vi "Test Platine newport.vi"() -> ()   [LabVIEW 2024]
uses:
  Newport.SMC100.CommandInterface
panel:
  in  "Init":bool
  out "Etat Controleur":bool
  out "StageIdentifier":string
  in  "Set Pos.Abs":bool
  in  "RESET Ctrl":bool
  in  "TargetPosition Abs":dbl
  out "Get PA Position":dbl
  out "Open Error":i32
  out "controllerState":string
  out "Close Error":i32
  in  "Controller address":i32=1
  out "CurrentPosition":dbl
  out "TS error":i32
  out "TP error":i32
  out "VE error":i32
  out "Error out":errorcluster caption="error out"
  in  "COM Port":string
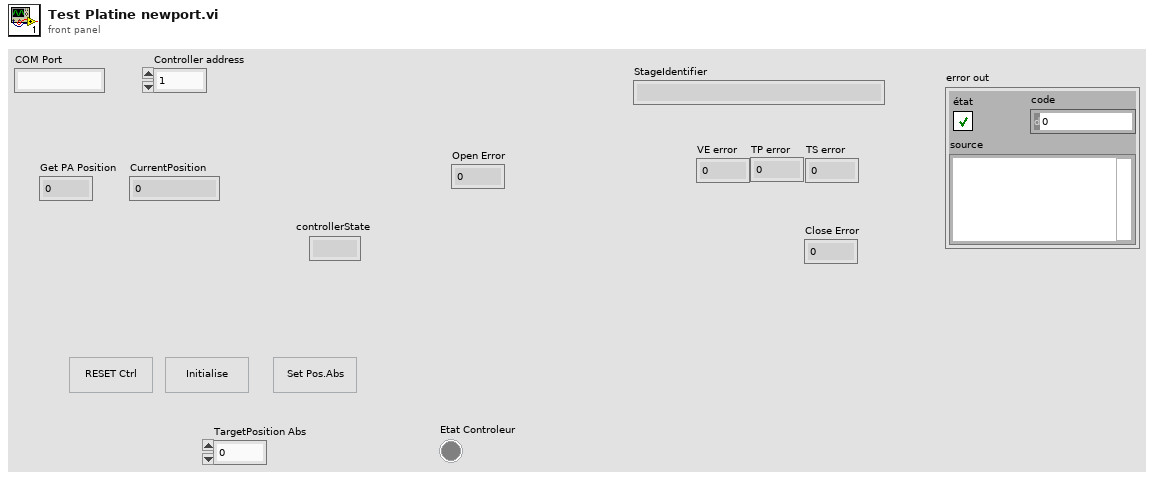
[diagram p1: front panel]
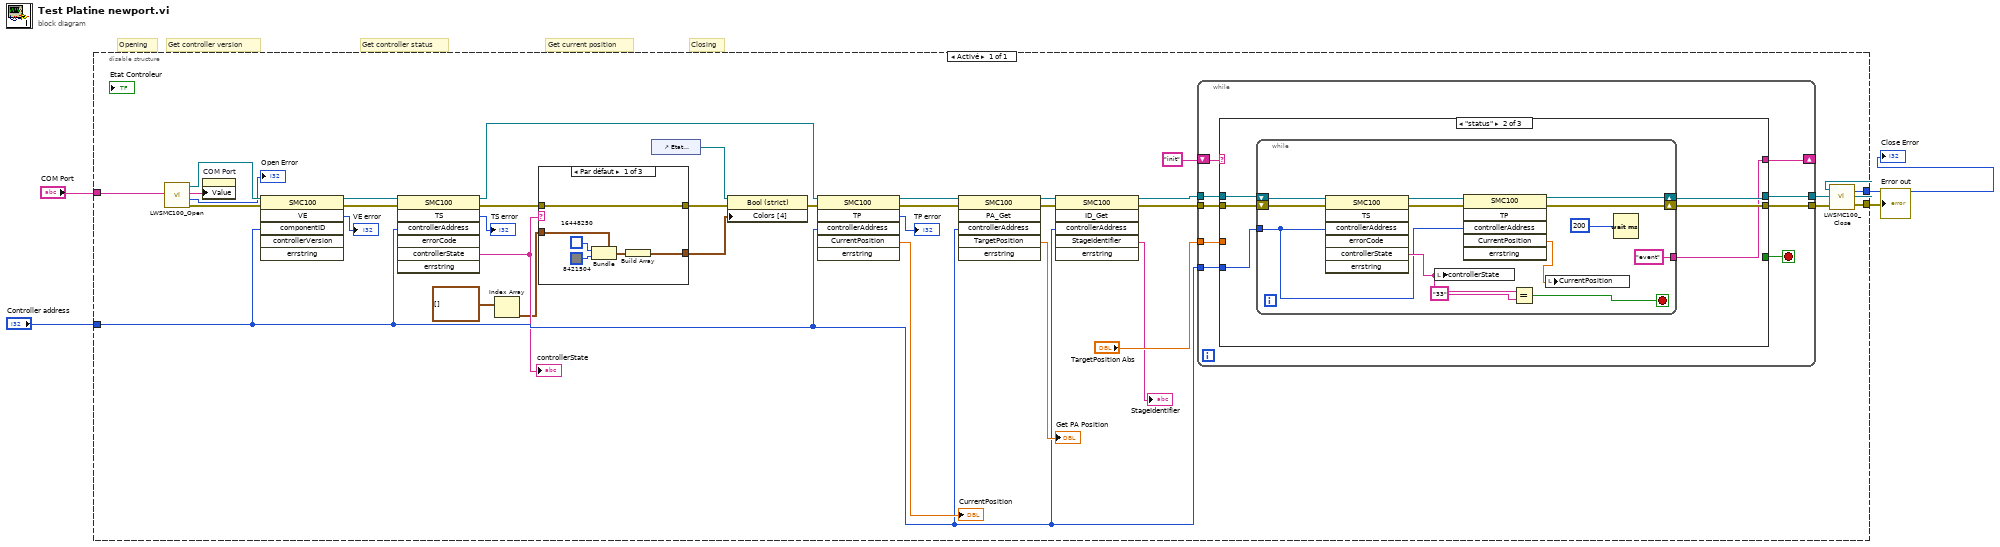
[diagram p0: block diagram]
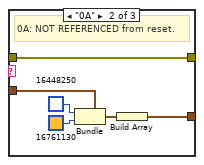
[diagram p2: hidden frame]
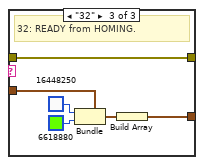
[diagram p3: hidden frame]
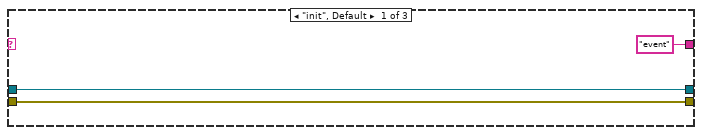
[diagram p4: hidden frame]
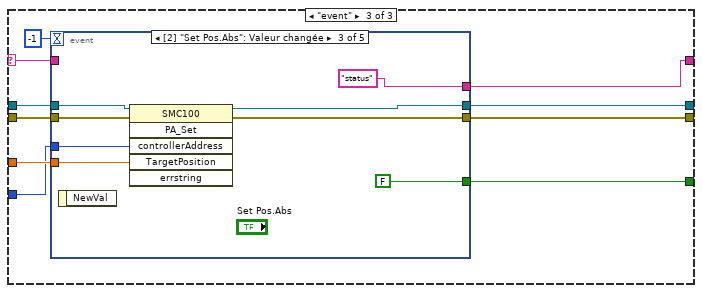
[diagram p5: hidden frame]
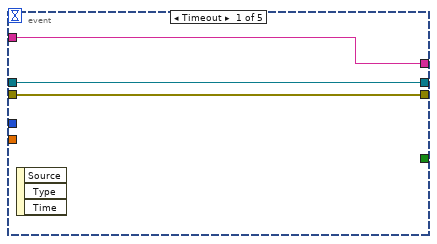
[diagram p6: hidden frame]
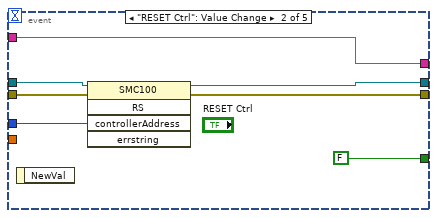
[diagram p7: hidden frame]
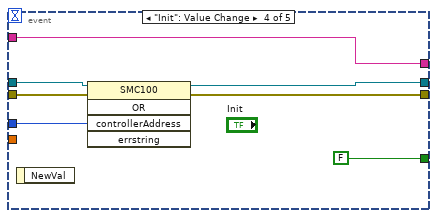
[diagram p8: hidden frame]
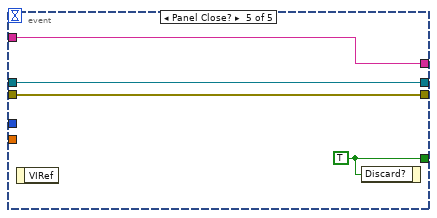
[diagram p9: hidden frame]
diagram:
  # "Get controller status"
  # "Get controller version"
  # "Get current position"
  # "Closing"
  # "Opening"
  n1 = disable-structure shown="Activé" {
    disable-tunnel: [w39] -> w4
    disable-tunnel: "COM Port" -> [w32]
    disable-tunnel: [w27] -> w2
    disable-tunnel: "Controller address" -> [w15]
    frame Enabled {
      n2 = call "LWSMC100_Open.vi"("Instrument Key IN"=w32) -> ("error out"=w31:errorcluster, "Error"=→"Open Error":i32, "Instrument Key OUT"=w33:string, "CommandInterfaceSMC100.SMC100"=w30:refnum<k24>)  [unwired: 3 in]
      n3 = property on="COM Port" class="Ch"("Value"=w33) -> ()  [unwired: 2 in, 2 out]
      n4 = invoke class="SMC100" method="VE"(reference=w30, error in=w31, "componentID"=w15) -> (reference out=w34:refnum<k24>, error out=w29:errorcluster, "VE"=→"VE error":i32)  [unwired: 3 in, 3 out]
      n5 = invoke class="SMC100" method="TS"(reference=w34, error in=w29, "controllerAddress"=w15) -> (reference out=w36:refnum<k24>, error out=w11:errorcluster, "TS"=→"TS error":i32, "controllerState"=w12:string)  [unwired: 4 in, 3 out]
      "controllerState" <- w12
      n6 = Index Array(array=cluster{u32, u32}[] [] ("Couls [4]")) -> (element=w9:cluster{u32, u32})  [unwired: 1 in]
      n7 = case shown="Par défaut" w12 {
        tunnel: w11 -> [w45 w51 w57]
        tunnel: [w45 w51 w57] -> w7
        tunnel: w9 -> [w41 w48 w54]
        tunnel: [w40 w46 w52] -> w8
        frame Default {
          n8 = Bundle(cluster=w41, u32 16448250, u32 8421504) -> (w42:cluster{u32, u32})
          n9 = Build Array(w42) -> (w40:cluster{u32, u32}[])
        }
        frame "0A" {
          # "0A: NOT REFERENCED from reset."
          n10 = Bundle(cluster=w48, u32 16448250, u32 16761130) -> (w47:cluster{u32, u32})
          n11 = Build Array(w47) -> (w46:cluster{u32, u32}[])
        }
        frame "32" {
          # "32: READY from HOMING."
          n12 = Bundle(cluster=w54, u32 16448250, u32 6618880) -> (w53:cluster{u32, u32})
          n13 = Build Array(w53) -> (w52:cluster{u32, u32}[])
        }
      }
      n14 = control-ref of="Etat Controleur"() -> (w13:refnum<vi>)
      n15 = property class="Bool (strict)"(reference=w13, error in=w7, "Colors [4]"=w8) -> (error out=w6:errorcluster)  [unwired: 1 out]
      n16 = invoke class="SMC100" method="TP"(reference=w36, error in=w6, "controllerAddress"=w15) -> (reference out=w24:refnum<k24>, error out=w25:errorcluster, "TP"=→"TP error":i32, "CurrentPosition"=→"CurrentPosition":dbl)  [unwired: 3 in, 2 out]
      n17 = invoke class="SMC100" method="PA_Get"(reference=w24, error in=w25, "controllerAddress"=w15) -> (reference out=w22:refnum<k24>, error out=w21:errorcluster, "TargetPosition"=→"Get PA Position":dbl)  [unwired: 3 in, 3 out]
      n18 = invoke class="SMC100" method="ID_Get"(reference=w22, error in=w21, "controllerAddress"=w15) -> (reference out=w19:refnum<k24>, error out=w20:errorcluster, "StageIdentifier"=→"StageIdentifier":string)  [unwired: 3 in, 3 out]
      n19 = while {
        tunnel: w19 -> [w66]
        tunnel: w20 -> [w65]
        tunnel: [w64] -> w18
        tunnel: [w63] -> w17
        tunnel: "TargetPosition Abs" -> [w62]
        tunnel: w15 -> [w60]
        shift-right: [w58] -> _
        shift-left: "init" -> [w59]
        stop <- w61 stop-if-true
        n20 = case shown="\"status\"" w59 {
          selector: w59 -> [_ _ w90]
          tunnel: w66 -> [w69 w75 w98]
          tunnel: w65 -> [w68 w73 w97]
          tunnel: [w68 w72 w96] -> w64
          tunnel: [w69 w74 w95] -> w63
          tunnel: w62 -> [_ _ w94]
          tunnel: [_ _ w93] -> w61
          tunnel: w60 -> [_ w71 w92]
          tunnel: ["event" w70 w91] -> w58
          frame "init", Default {
          }
          frame "status" {
            n21 = while {
              tunnel: w71 -> [w77]
              shift-right: [w79] -> w74
              shift-left: w75 -> [w88]
              shift-right: [w80] -> w72
              shift-left: w73 -> [w87]
              tunnel: ["event"] -> w70
              stop <- w85 stop-if-true
              n22 = invoke class="SMC100" method="TS"(reference=w88, error in=w87, "controllerAddress"=w77) -> (reference out=w78:refnum<k24>, error out=w81:errorcluster, "controllerState"=w82:string)  [unwired: 4 in, 4 out]
              n23 = local write "controllerState"(w82) -> ()
              n24 = invoke class="SMC100" method="TP"(reference=w78, error in=w81, "controllerAddress"=w77) -> (reference out=w79:refnum<k24>, error out=w80:errorcluster, "CurrentPosition"=w76:dbl)  [unwired: 3 in, 3 out]
              n25 = Equal?(x=w82, y="33") -> (x = y?=w85:bool)
              n26 = local write "CurrentPosition"(w76) -> ()
              n27 = Wait (ms)(milliseconds to wait=u32 200 ("attente (ms)")) -> ()  [unwired: 1 out]
            }
          }
          frame "event" {
            n28 = event shown="[2] \"Set Pos.Abs\": Valeur changée" {
              selector: _ -> [_ _ _ _ _]
              dyn-events: _ -> [_ _ _ _ _]
              timeout: -1 -> [_ _ _ _ _]
              tunnel: w98 -> [w101 w108 w116 w122 w125]
              tunnel: w97 -> [w100 w107 w113 w119 w126]
              tunnel: [w100 w106 w114 w120 w126] -> w96
              tunnel: [w101 w105 w115 w121 w125] -> w95
              tunnel: w94 -> [_ _ w112 _ _]
              tunnel: [_ FALSE FALSE ("Rejeter ?") FALSE ("Rejeter ?") w127] -> w93
              tunnel: w92 -> [_ w104 w111 w118 _]
              tunnel: [w99 w102 "status" w117 w124] -> w91
              tunnel: w90 -> [w99 w102 _ w117 w124]
              event Timeout {
                n29 = event-data() -> ()  [unwired: 1 in, 3 out]
              }
              event "RESET Ctrl": Value Change {
                n30 = event-data() -> ()  [unwired: 1 in, 1 out]
                n31 = invoke class="SMC100" method="RS"(reference=w108, error in=w107, "controllerAddress"=w104) -> (reference out=w105:refnum<k24>, error out=w106:errorcluster)  [unwired: 2 in, 3 out]
              }
              event "Set Pos.Abs": Value Change {
                n32 = event-data() -> ()  [unwired: 1 in, 1 out]
                n33 = invoke class="SMC100" method="PA_Set"(reference=w116, error in=w113, "controllerAddress"=w111, "TargetPosition"=w112) -> (reference out=w115:refnum<k24>, error out=w114:errorcluster)  [unwired: 2 in, 4 out]
              }
              event "Init": Value Change {
                n34 = event-data() -> ()  [unwired: 1 in, 1 out]
                n35 = invoke class="SMC100" method="OR"(reference=w122, error in=w119, "controllerAddress"=w118) -> (reference out=w121:refnum<k24>, error out=w120:errorcluster)  [unwired: 2 in, 3 out]
              }
              event Panel Close? {
                w127 = TRUE ("Rejeter ?")
                n36 = event-data() -> ()  [unwired: 1 in, 1 out]
                n37 = event-data("Discard?"=w127) -> ()  [unwired: 1 in, 1 out]
              }
            }
          }
        }
      }
      n38 = call "LWSMC100_Close.vi"("error in (no error)"=w18, "CommandInterfaceSMC100.SMC100"=w17) -> ("Error out"=w39:errorcluster, "Error"=w27:i32)  [unwired: 1 in]
    }
  }
  "Error out" <- w4
  "Close Error" <- w2
